vi "Create Events.vi"(0 "Display State In":T2, 9 "Container State":T6, 11 "error in (no error)":errorcluster) -> (4 "Display State Out":T2, 8 "Events":T1, 15 "error out":errorcluster)   [LabVIEW 2015, in "Interactive Graph.xctl"]
uses:
  Interactive Graph.xctl
  <vilib>/_xctls/Container State.ctl
  State.vi
  Persistent.ctl
  Plot.ctl
  EPhys/LV Source/Work Panel VIs/Typedefs/EPhysWork-Label Position.ctl
  Events.ctl
  Selection.ctl
  XRange.ctl
  YScale.ctl
  Cursor.ctl
  <vilib>/_xctls/XControlSupport.lvlib
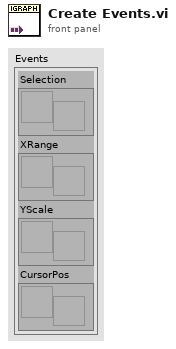
[diagram p1: front panel]
types:
  T1 = typedef "Interactive Graph.xctl/Events.ctl" = cluster{"Selection":refnum<user-event>, "XRange":refnum<user-event>, "YScale":refnum<user-event>, "CursorPos":refnum<user-event>}
  T2 = typedef "Interactive Graph.xctl/State.vi" = cluster{"ref":refnum<vi>, "actions":string[], "Persist":T3, "cursor":bool, "prescale":dbl, "palette":u32[], "colIndex":i32, "to add":T4, "Events":T1, "selected":i32, "to show":cluster{"Visible":bool, "Start":i32, "Length":i32}, "maxplot":i32, "Y0":dbl[], "plotnum":i32, "length":i32}
  T3 = typedef "Interactive Graph.xctl/Persistent.ctl" = cluster{"Scale":dbl, "Xrange":cluster{"min":dbl, "max":dbl}}
  T4 = typedef "Interactive Graph.xctl/Plot.ctl" = cluster{"plot":cluster{"X":dbl[], "Y":dbl[]}, "name":string, "Y0":dbl, "color":u32, "Style":enum16{"Normal", "Highlight", "Shadow"}, "labpos":T5, "visible":bool, "cursor":bool}
  T5 = typedef "EPhysWork-Label Position.ctl" = cluster{"Index":i32, "Xoff":dbl, "Yoff":dbl}
  T6 = typedef "XControlSupport.lvlib/Container State.ctl" = cluster{"Indicator?":bool, "Run Mode?":bool, " Refnum":refnum<vi>}
  T7 = typedef "Interactive Graph.xctl/Cursor.ctl" = cluster{"X":dbl, "Y":dbl}
  T8 = typedef "Interactive Graph.xctl/YScale.ctl" = cluster{"Value":dbl}
  T9 = typedef "Interactive Graph.xctl/XRange.ctl" = cluster{"Min":dbl, "Max":dbl}
  T10 = typedef "Interactive Graph.xctl/Selection.ctl" = cluster{"Value":i32}
  T11 = cluster{"Event Data":refnum<user-event>, "Event Data":refnum<user-event>, "Event Data":refnum<user-event>, "Event Data":refnum<user-event>}
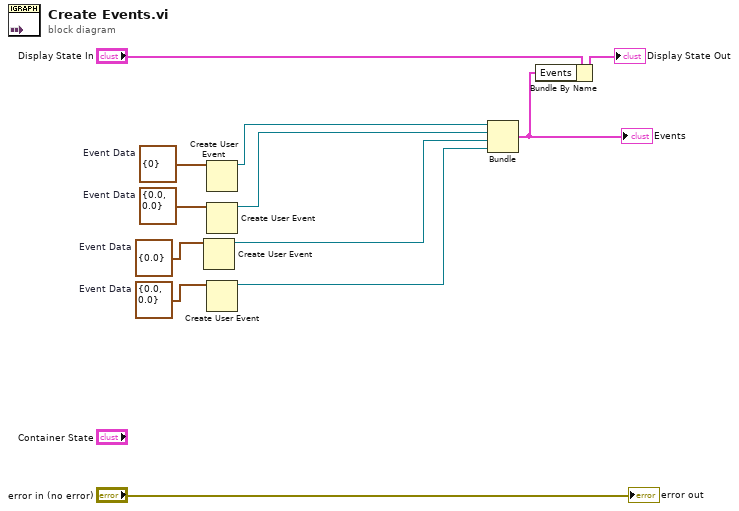
[diagram p0: block diagram]
diagram:
  w3 = T7 {"X"=0.0, "Y"=0.0}  # Event Data
  w5 = T8 {"Value"=0.0}  # Event Data
  w7 = T9 {"Min"=0.0, "Max"=0.0}  # Event Data
  w8 = T10 {"Value"=0}  # Event Data
  n1 = Create User Event(user event datatype=w5) -> (user event=w4:refnum<user-event>)  [unwired: 1 in, 1 out]
  n2 = Create User Event(user event datatype=w8) -> (user event=w9:refnum<user-event>)  [unwired: 1 in, 1 out]
  n3 = Create User Event(user event datatype=w7) -> (user event=w6:refnum<user-event>)  [unwired: 1 in, 1 out]
  n4 = Create User Event(user event datatype=w3) -> (user event=w2:refnum<user-event>)  [unwired: 1 in, 1 out]
  n5 = Bundle("Event Data"=w9, "Event Data"=w6, "Event Data"=w4, "Event Data"=w2) -> (w1:T11)  [unwired: 1 in]
  "Events" <- w1
  n6 = Bundle By Name(cluster="Display State In", "Events"=w1) -> (→"Display State Out":T2)
  "error out" <- "error in (no error)"
